vi "CreateObject.vi"(8 "ErrorIn":errorcluster, 10 "ObjectName":string, 11 "Type":refnum<class>) -> (0 "ErrorOut":errorcluster, 3 "ObjectOut":refnum<class>)   [LabVIEW 2021, in "Application.lvclass"]
uses:
  Application.lvclass
  Interface_TAF_ITAFObject/ITAFObject/ITAFObject.lvclass
  b3bde5ba-cb20-4692-bd91-ec82fe1b2db2.vi
  <vilib>/TriekselSoft/TracerLibrary/TracerLibrary/Tracer/protected/SendMessage.vi
  <vilib>/TriekselSoft/TracerLibrary/TracerLibrary/Tracer/protected/Timestamp.vi
  b3bde5ba-cb20-4692-bd91-ec82fe1b2db2.vi/f75db090-0877-4668-94fb-75c2140b1617.vi
  <vilib>/TriekselSoft/TracerLibrary/TracerLibrary/Tracer/Tracer_Level-Debug.vi
  <vilib>/JDP Science/JSONtext/Variant to JSON Text.vi
  <vilib>/TriekselSoft/TracerLibrary/TracerLibrary/Tracer/protected/Tracer_ClassAttributes.vi
  <vilib>/JDP Science/JSONtext/LVClass Serializer/JSONtext LVClass Serializer.lvclass
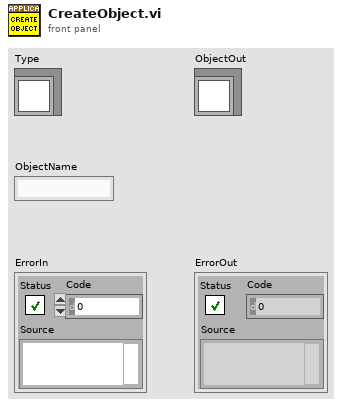
[diagram p1: front panel]
types:
  T1 = typedef "Application.lvclass/ObjectAttributes.ctl" = cluster{"Objects":variant, "BasePath":path, "Application":refnum<class "Application.lvclass">}
  T2 = cluster{"ObjectName":string, "class name":string}
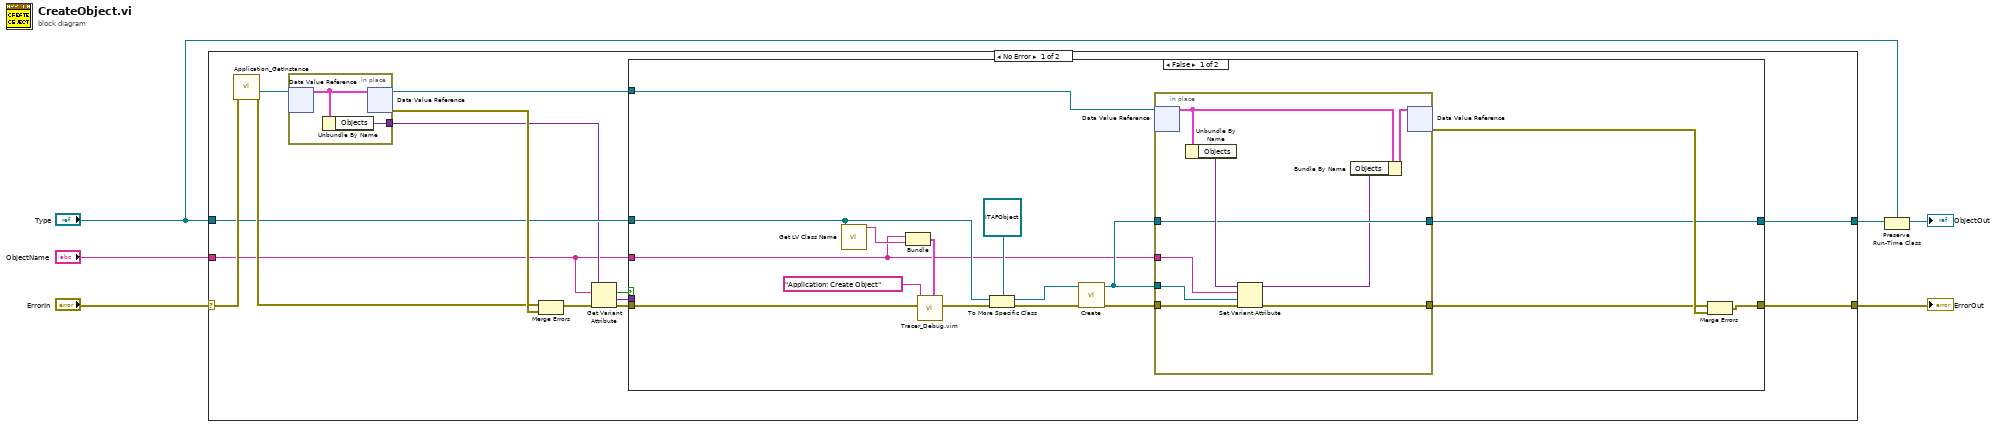
[diagram p0: block diagram]
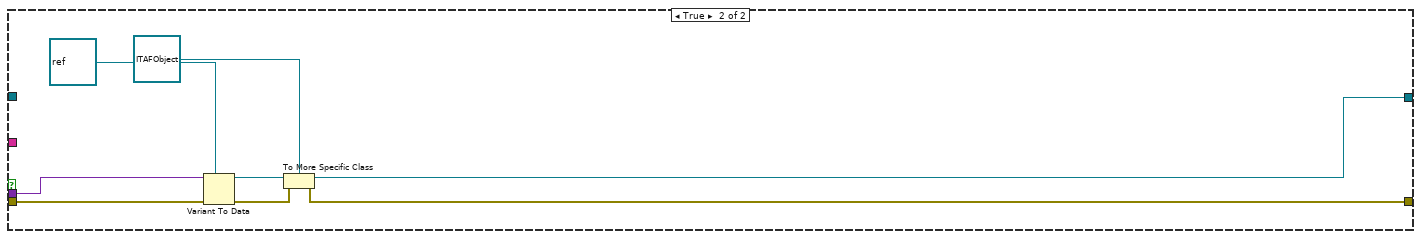
[diagram p2: hidden frame]
diagram:
  n1 = case shown="No Error" "ErrorIn" {
    selector: "ErrorIn" -> [w20 w57]
    tunnel: [w16 w57] -> w5
    tunnel: "ObjectName" -> [w7 _]
    tunnel: "Type" -> [w14 _]
    tunnel: [w13 _] -> w3
    frame No Error {
      n2 = call "Application_GetInstance.vi"("ErrorIn"=w20) -> ("ErrorOut"=w15:errorcluster, "DVRRefOut"=w12:refnum<data-value>)  [unwired: 6 in, 3 out]
      n3 = in-place {
        in-place-border: [w55] -> w9
        n4 = in-place-dvr #1(w12) -> (w56:T1)  [unwired: 1 out]
        n5 = Unbundle By Name(w56) -> ("Objects"=w55:variant)
        n6 = in-place-dvr #1(w56) -> (w8:refnum<data-value>, w19:errorcluster)
      }
      n7 = Merge Errors(w15, w19) -> (w18:errorcluster)
      n8 = Get Variant Attribute(Variant=w9, name=w7, error in=w18) -> (found=w11:bool, value=w10:variant, error out=w17:errorcluster)  [unwired: 1 in, 1 out]
      n9 = case shown="False" w11 {
        tunnel: w17 -> [w31 w54]
        tunnel: w14 -> [w25 _]
        tunnel: [w37 w52] -> w16
        tunnel: [w21 w47] -> w13
        tunnel: w10 -> [_ w50]
        tunnel: w8 -> [w30 _]
        tunnel: w7 -> [w22 _]
        frame False {
          n10 = call <vilib>:"Get LV Class Name.vi"("object"=w25) -> ("class name"=w24:string)  [unwired: 9 in, 1 out]
          n11 = Bundle("ObjectName"=w22, "class name"=w24) -> (w23:T2)  [unwired: 1 in]
          n12 = call "Tracer_Debug.vim"("Data"=w23, "Error In"=w31, "Text"="Application: Create Object") -> ("Error Out"=w33:errorcluster)  [unwired: 8 in]
          n13 = To More Specific Class(target class=refnum<class "ITAFObject.lvclass"> refnum ("ClassActor"), reference=w25, error in=w33) -> (specific class reference=w28:refnum<class "ITAFObject.lvclass">, error out=w35:errorcluster)
          n14 = call-dynamic "Create.vi"("ErrorIn"=w35, "ObjectIn"=w28) -> ("ErrorOut"=w34:errorcluster, "ObjectOut"=w27:refnum<class "ITAFObject.lvclass">)  [unwired: 8 in]
          n15 = in-place {
            in-place-border: w27 -> [w39]
            in-place-border: w22 -> [w40]
            in-place-border: w34 -> [w46]
            in-place-border: [w45] -> w32
            in-place-border: [w41] -> w21
            in-place-border: w27 -> [w41]
            n16 = in-place-dvr #2(w30) -> (w44:T1)  [unwired: 1 out]
            n17 = Unbundle By Name(w44) -> ("Objects"=w42:variant)
            n18 = Set Variant Attribute(Variant=w42, name=w40, value=w39, error in=w46) -> (Variant out=w38:variant, error out=w45:errorcluster)  [unwired: 1 out]
            n19 = Bundle By Name(cluster=w44, "Objects"=w38) -> (w43:T1)
            n20 = in-place-dvr #2(w43) -> (w36:errorcluster)  [unwired: 1 out]
          }
          n21 = Merge Errors(w32, w36) -> (w37:errorcluster)
        }
        frame True {
          n22 = Variant To Data(error in=w54, type=refnum<class> refnum ("Type"), Variant=w50) -> (data=w48:refnum<class>, error out=w53:errorcluster)
          n23 = To More Specific Class(target class=refnum<class "ITAFObject.lvclass"> refnum ("ClassActor"), reference=w48, error in=w53) -> (specific class reference=w47:refnum<class "ITAFObject.lvclass">, error out=w52:errorcluster)
        }
      }
    }
    frame Error {
    }
  }
  "ErrorOut" <- w5
  n24 = Preserve Run-Time Class(object in=w3, 2:"Type") -> (object out=→"ObjectOut":refnum<class>)  [unwired: 1 in, 1 out]
